vi "ClientForSingleDeviceDServer_03.vi"() -> ()   [LabVIEW 2014, in "examples.lvlib"]
uses:
  examples.lvlib
  Common/UtilsRandomInstances/_UtilsRandomI16Array.vi
  vis/tango_vi.llb/WriteShortSpectrumAttribute.vi
  vis/tango_vi.llb/ReadShortSpectrumAttribute.vi
  Common/UtilsRandomInstances/_UtilsRandomU16Array.vi
  vis/tango_vi.llb/WriteUShortSpectrumAttribute.vi
  vis/tango_vi.llb/ReadUShortSpectrumAttribute.vi
  Common/UtilsRandomInstances/_UtilsRandomBoolArray.vi
  vis/tango_vi.llb/WriteBooleanSpectrumAttribute.vi
  vis/tango_vi.llb/ReadBooleanSpectrumAttribute.vi
  Common/UtilsRandomInstances/_UtilsRandomU8Array.vi
  vis/tango_vi.llb/WriteUCharSpectrumAttribute.vi
  vis/tango_vi.llb/ReadUCharSpectrumAttribute.vi
  Common/UtilsRandomInstances/_UtilsRandom2DI16Array.vi
  vis/tango_vi.llb/WriteShortImageAttribute.vi
  vis/tango_vi.llb/ReadShortImageAttribute.vi
  Common/UtilsRandomInstances/_UtilsRandomSGLArray.vi
  vis/tango_vi.llb/WriteFloatSpectrumAttribute.vi
  vis/tango_vi.llb/ReadFloatSpectrumAttribute.vi
  Common/UtilsRandomInstances/_UtilsRandomDBLArray.vi
  vis/tango_vi.llb/WriteDoubleSpectrumAttribute.vi
  vis/tango_vi.llb/ReadDoubleSpectrumAttribute.vi
  Common/UtilsRandomInstances/_UtilsRandom2DI32Array.vi
  vis/tango_vi.llb/WriteLongImageAttribute.vi
  vis/tango_vi.llb/ReadLongImageAttribute.vi
  Common/UtilsRandomInstances/_UtilsRandomU32Array.vi
  vis/tango_vi.llb/WriteLongSpectrumAttribute.vi
  vis/tango_vi.llb/ReadLongSpectrumAttribute.vi
  Common/UtilsRandomInstances/_UtilsRandom2DU16Array.vi
  vis/tango_vi.llb/WriteUShortImageAttribute.vi
  vis/tango_vi.llb/ReadUShortImageAttribute.vi
  Common/UtilsRandomInstances/_UtilsRandom2DU8Array.vi
  vis/tango_vi.llb/WriteUCharImageAttribute.vi
  vis/tango_vi.llb/ReadUCharImageAttribute.vi
  Common/UtilsRandomInstances/_UtilsRandom2DBoolArray.vi
  vis/tango_vi.llb/WriteBooleanImageAttribute.vi
  vis/tango_vi.llb/ReadBooleanImageAttribute.vi
  Common/UtilsRandomInstances/_UtilsRandom2DSGLArray.vi
  vis/tango_vi.llb/WriteFloatImageAttribute.vi
  vis/tango_vi.llb/ReadFloatImageAttribute.vi
  Common/UtilsRandomInstances/_UtilsRandom2DDBLArray.vi
  vis/tango_vi.llb/WriteDoubleImageAttribute.vi
  vis/tango_vi.llb/ReadDoubleImageAttribute.vi
  Common/UtilsRandomInstances/_UtilsRandom2DU32Array.vi
  vis/tango_vi.llb/WriteULongImageAttribute.vi
  vis/tango_vi.llb/ReadULongImageAttribute.vi
  vis/tango_vi.llb/tango.lvlib
panel:
  out "Success-R":bool
  out "Success-Comp":bool
  out "devULongImage R":u32[][](graph)
  out "Success-W":bool
  out "devULongImage W":u32[][](graph)
  out "Success-R":bool
  out "Success-Comp":bool
  out "devDoubleImage R":dbl[][](graph)
  out "Success-W":bool
  out "devDoubleImage W":dbl[][](graph)
  out "Success-R":bool
  out "Success-Comp":bool
  out "devFloatImage R":sgl[][](graph)
  out "Success-W":bool
  out "devFloatImage W":sgl[][](graph)
  out "Success-R":bool
  out "Success-Comp":bool
  out "devBooleanImage R":i16[][](graph)
  out "Success-W":bool
  out "devBooleanImage W":i16[][](graph)
  out "Success-R":bool
  out "Success-Comp":bool
  out "devUCharImage R":u8[][](graph)
  out "Success-W":bool
  out "devUCharImage W":u8[][](graph)
  out "Success-R":bool
  out "Success-Comp":bool
  out "devUShortImage R":u16[][](graph)
  out "Success-W":bool
  out "devUShortImage W":u16[][](graph)
  out "devLongSpectrum R":i32[](graph)
  out "Success-R":bool
  out "Success-Comp":bool
  out "Success-W":bool
  out "devLongSpectrum W":i32[](graph)
  out "Success-R":bool
  out "Success-Comp":bool
  out "devLongImage R":i32[][](graph)
  out "Success-W":bool
  out "devLongImage W":i32[][](graph)
  out "devDoubleSpectrum R":dbl[](graph)
  out "Success-R":bool
  out "Success-Comp":bool
  out "Success-W":bool
  out "devDoubleSpectrum  W":dbl[](graph)
  out "devFloatSpectrum R":sgl[](graph)
  out "Success-R":bool
  out "Success-Comp":bool
  out "Success-W":bool
  out "devFloatSpectrum W":sgl[](graph)
  out "devShortImage R":i16[][](graph)
  out "devShortImage W":i16[][](graph)
  out "Success-R":bool
  out "Success-Comp":bool
  out "Success-W":bool
  in  "TangoTest Device Name 5":string="tango/tangotest/1"
  in  "TangoTest Device Name 4":string="tango/tangotest/1"
  in  "TangoTest Device Name 3":string="tango/tangotest/1"
  in  "TangoTest Device Name 2":string="tango/tangotest/1"
  in  "TangoTest dev. name":string="labview/device/1"
  out "devUCharSpectrum R":u8[](graph)
  out "Success-R":bool
  out "Success-Comp":bool
  out "Success-W":bool
  out "devUCharSpectrum W":u8[](graph)
  out "devBooleanSpectrum R":i16[](graph)
  out "Success-R":bool
  out "Success-Comp":bool
  out "Success-W":bool
  out "devBooleanSpectrum W":i16[](graph)
  out "devUShortSpectrum R":u16[](graph)
  out "Success-R":bool
  out "Success-Comp":bool
  out "Success-W":bool
  out "devUShortSpectrum W":u16[](graph)
  out "Success-Comp":bool
  out "Success-W":bool
  out "devShortSpectrum R":i16[](graph)
  out "Success-R":bool
  out "devShortSpectrum W":i16[](graph)
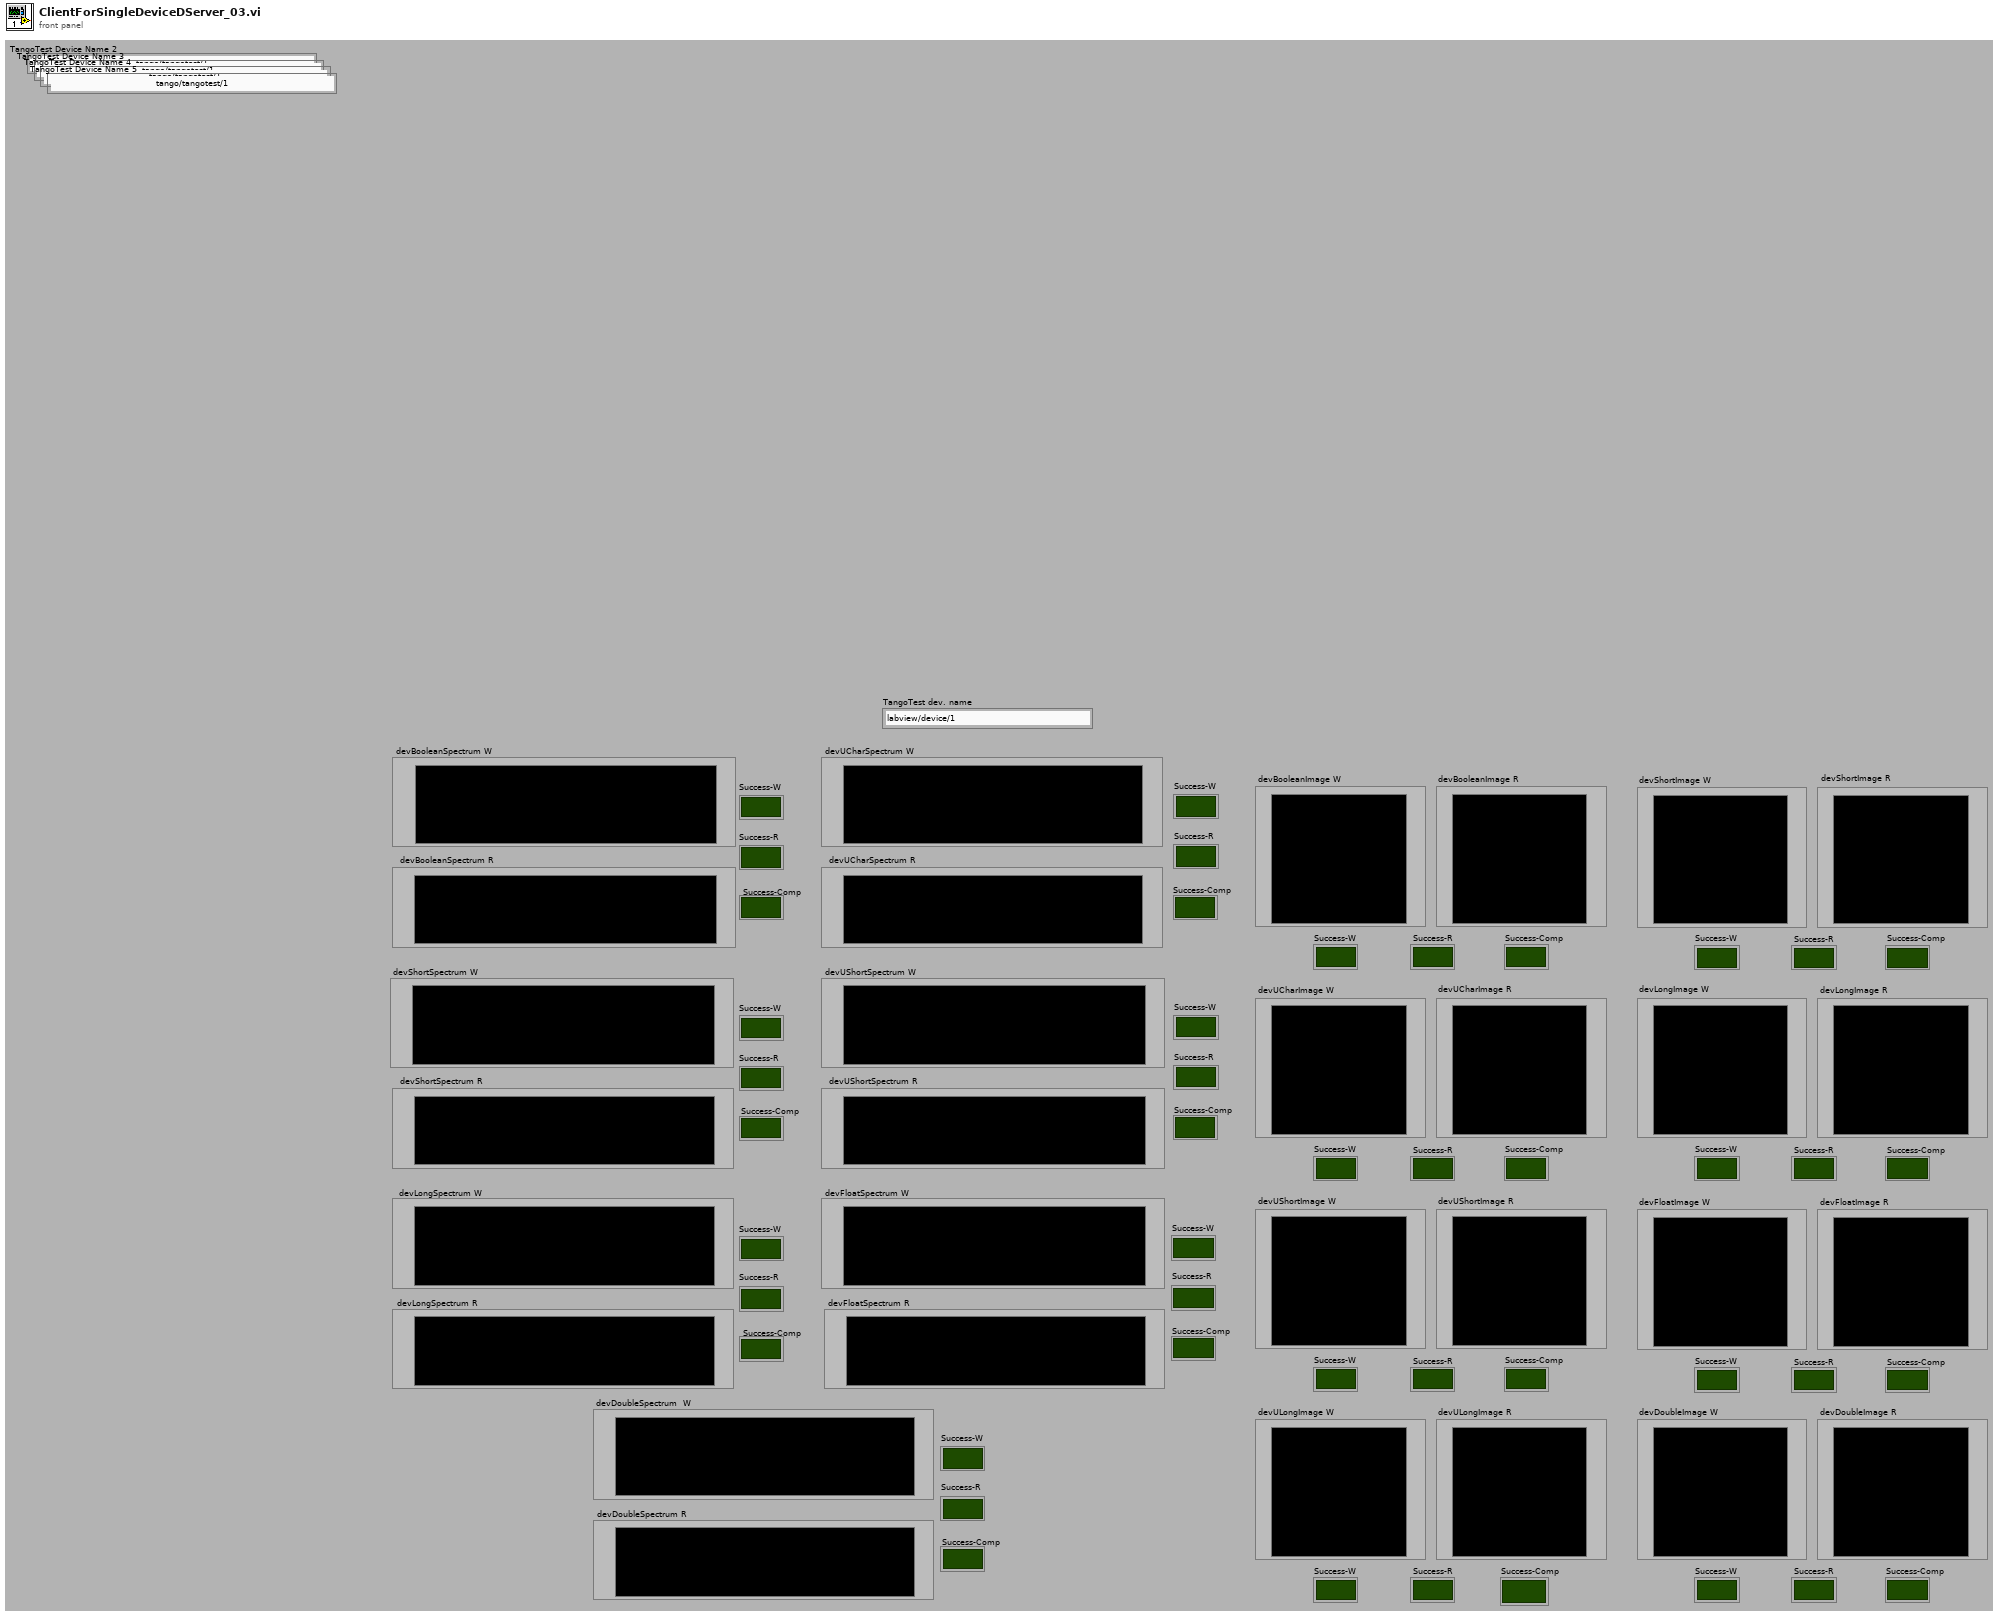
[diagram p1: front panel]
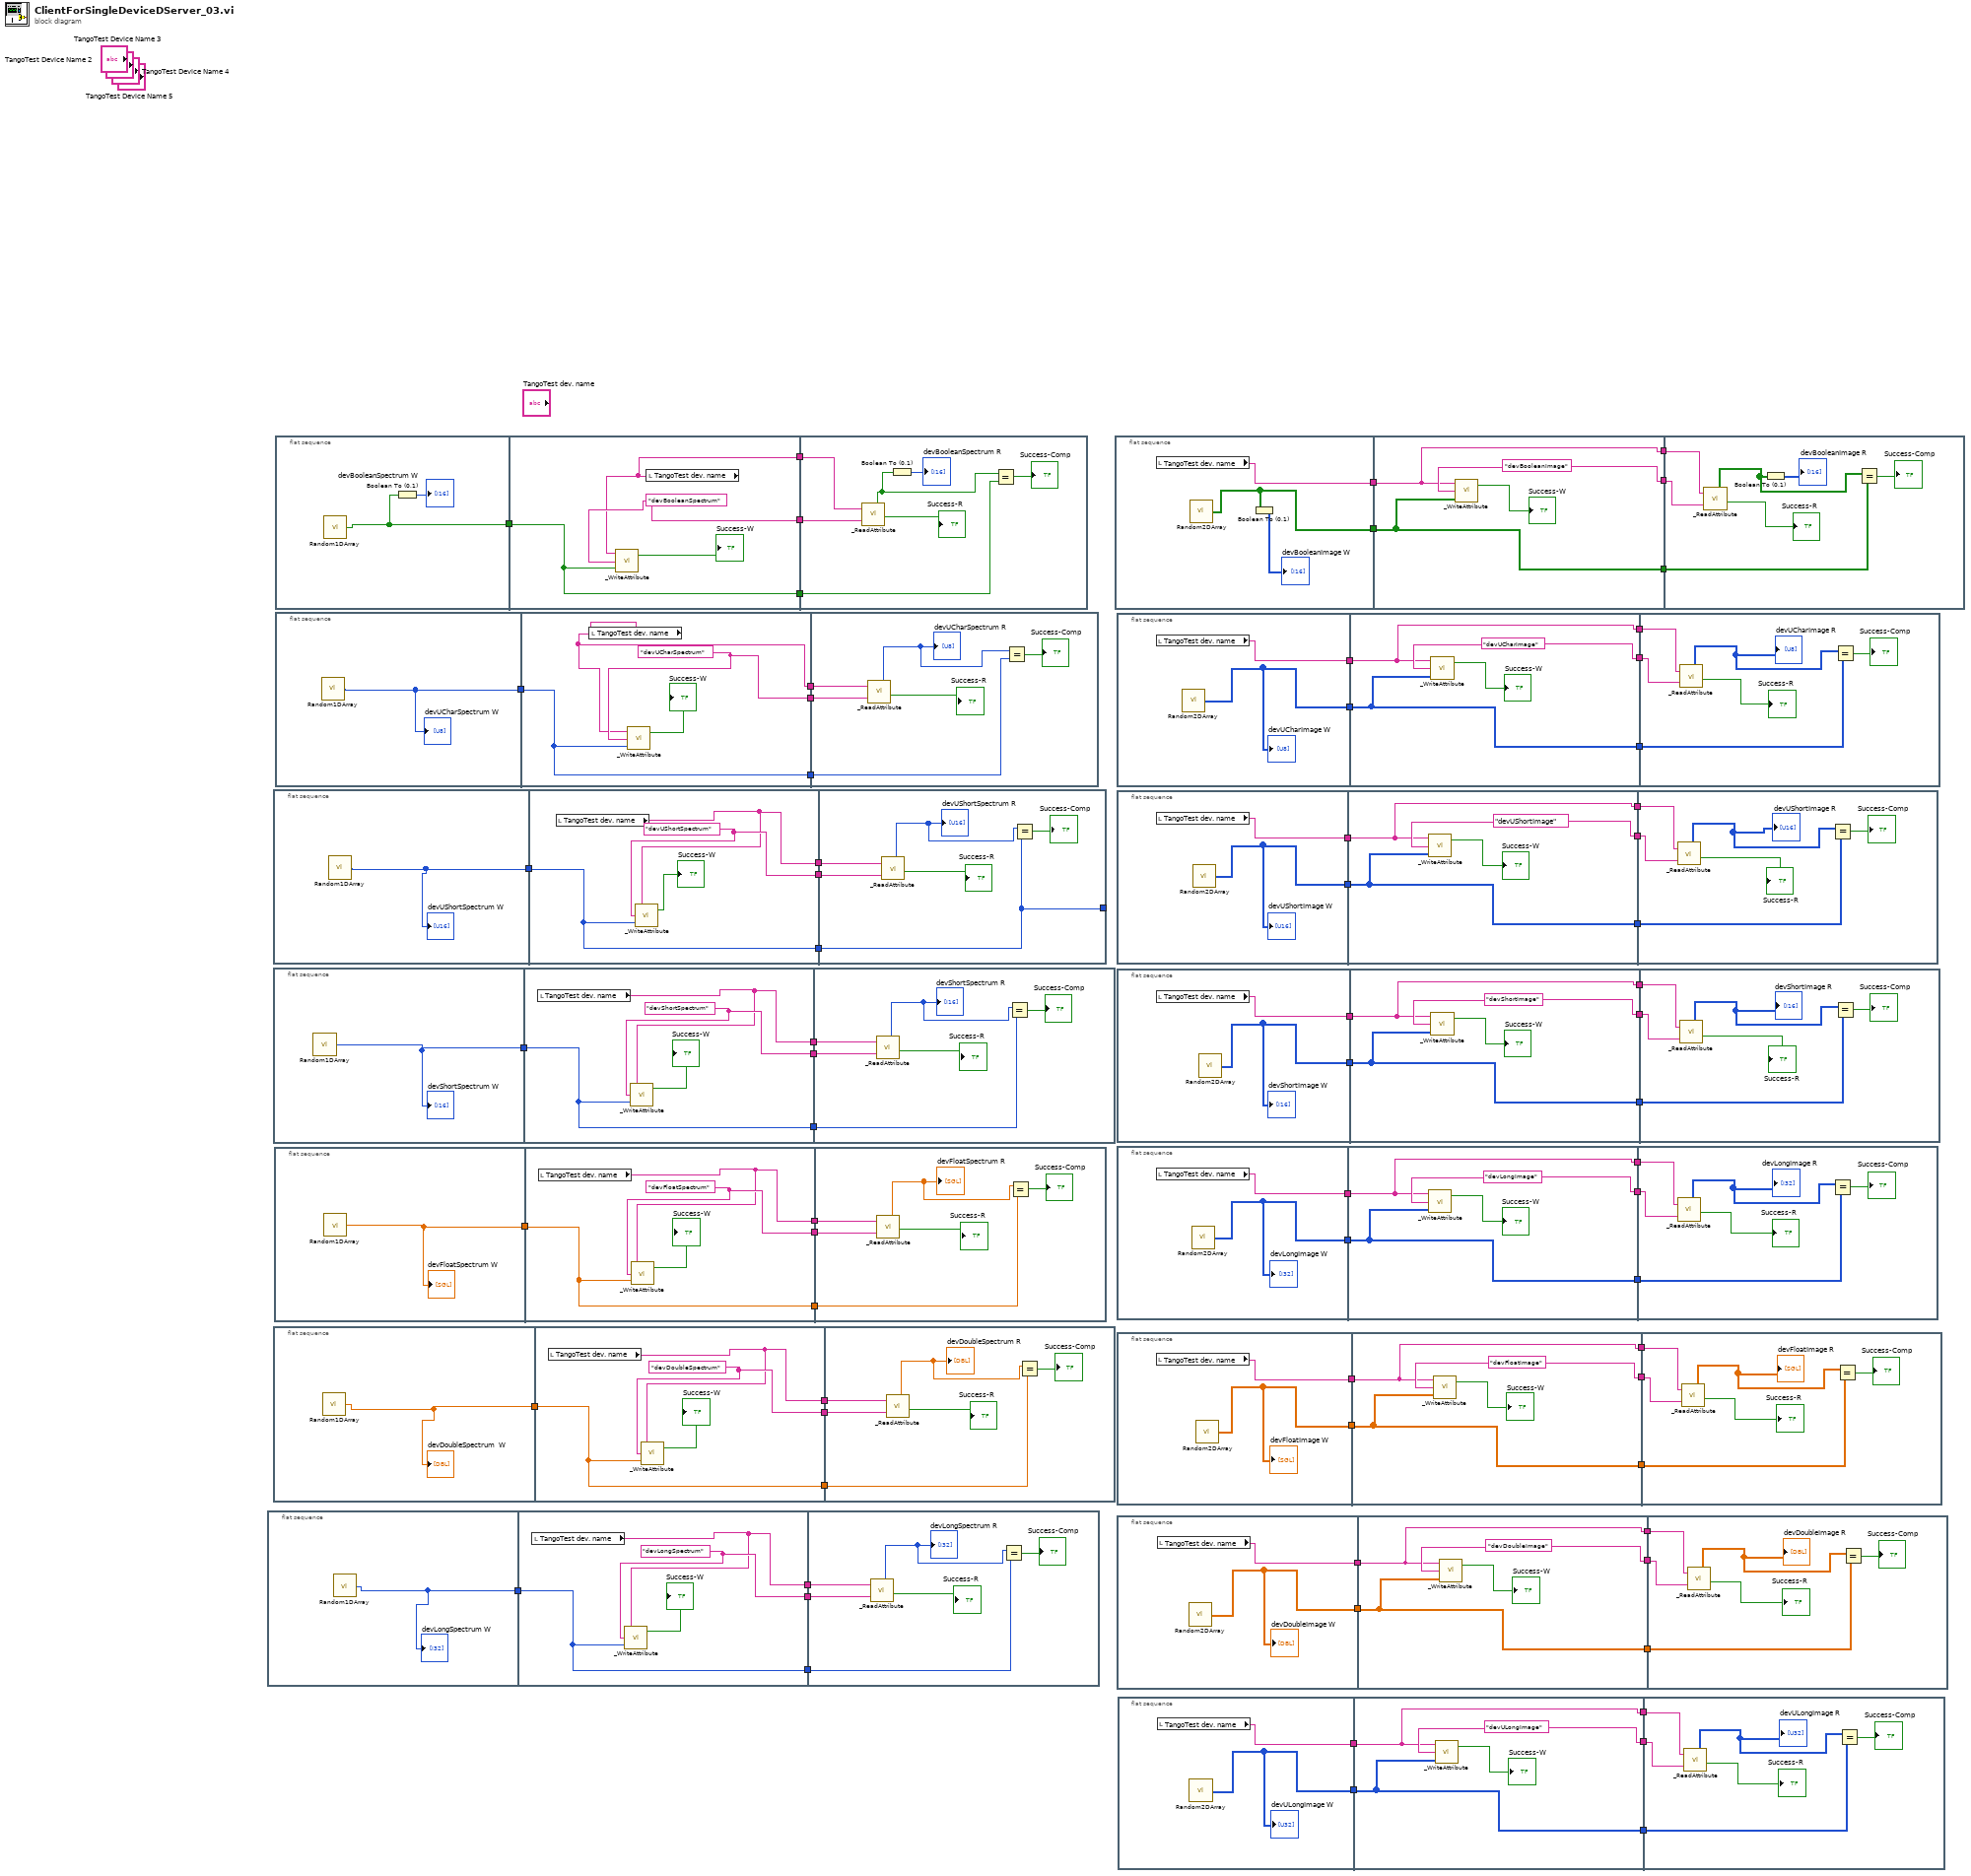
[diagram p0: block diagram]
diagram:
  n1 = flat-sequence {
    tunnel: [w69] -> w34
    tunnel: [w70] -> w33
    tunnel: [w72] -> w32
    tunnel: [w71] -> w31
    tunnel: w34 -> [w71]
    tunnel: w33 -> [w78]
    tunnel: w32 -> [w77]
    tunnel: w31 -> [w75]
    frame #0 {
      n2 = call-poly "Random1DArray.vi"() -> ("array"=w69:i32[])  [unwired: 2 in]
      "devLongSpectrum W" <- w69
    }
    frame #1 {
      w72 = "devLongSpectrum" ("attribute name")
      n3 = local read "TangoTest dev. name"() -> (w70:string)
      n4 = call-poly "_WriteAttribute.vi"("value"=w71, "attribute name"=w72, "device name"=w70) -> ("success"=→"Success-W":bool)  [unwired: 1 out]
    }
    frame #2 {
      n5 = call-poly "_ReadAttribute.vi"("device name"=w78, "attribute name"=w77) -> ("value"=w76:i32[], "success"=→"Success-R":bool)  [unwired: 4 out]
      "devLongSpectrum R" <- w76
      n6 = Equal?(x=w76, y=w75) -> (x = y?=→"Success-Comp":bool)
    }
  }
  n7 = flat-sequence {
    tunnel: [w80] -> w64
    tunnel: [w82] -> w63
    tunnel: [w84] -> w62
    tunnel: [w83] -> w61
    tunnel: w64 -> [w83]
    tunnel: w63 -> [w89]
    tunnel: w62 -> [w88]
    tunnel: w61 -> [w85]
    tunnel: [w85] -> _
    frame #0 {
      n8 = call-poly "Random1DArray.vi"() -> ("array"=w80:u16[])  [unwired: 2 in]
      "devUShortSpectrum W" <- w80
    }
    frame #1 {
      w84 = "devUShortSpectrum" ("attribute name")
      n9 = local read "TangoTest dev. name"() -> (w82:string)
      n10 = call-poly "_WriteAttribute.vi"("value"=w83, "attribute name"=w84, "device name"=w82) -> ("success"=→"Success-W":bool)  [unwired: 1 out]
    }
    frame #2 {
      n11 = call-poly "_ReadAttribute.vi"("device name"=w89, "attribute name"=w88) -> ("value"=w87:u16[], "success"=→"Success-R":bool)  [unwired: 4 out]
      "devUShortSpectrum R" <- w87
      n12 = Equal?(x=w87, y=w85) -> (x = y?=→"Success-Comp":bool)
    }
  }
  n13 = flat-sequence {
    tunnel: [w91] -> w65
    tunnel: [w92] -> w68
    tunnel: [w94] -> w67
    tunnel: [w93] -> w66
    tunnel: w65 -> [w93]
    tunnel: w68 -> [w100]
    tunnel: w67 -> [w99]
    tunnel: w66 -> [w97]
    frame #0 {
      n14 = call-poly "Random1DArray.vi"() -> ("array"=w91:i16[])  [unwired: 2 in]
      "devShortSpectrum W" <- w91
    }
    frame #1 {
      w94 = "devShortSpectrum" ("attribute name")
      n15 = local read "TangoTest dev. name"() -> (w92:string)
      n16 = call-poly "_WriteAttribute.vi"("value"=w93, "attribute name"=w94, "device name"=w92) -> ("success"=→"Success-W":bool)  [unwired: 1 out]
    }
    frame #2 {
      n17 = call-poly "_ReadAttribute.vi"("device name"=w100, "attribute name"=w99) -> ("value"=w98:i16[], "success"=→"Success-R":bool)  [unwired: 4 out]
      "devShortSpectrum R" <- w98
      n18 = Equal?(x=w98, y=w97) -> (x = y?=→"Success-Comp":bool)
    }
  }
  n19 = flat-sequence {
    tunnel: [w102] -> w43
    tunnel: [w103] -> w42
    tunnel: [w105] -> w41
    tunnel: [w104] -> w40
    tunnel: w43 -> [w104]
    tunnel: w42 -> [w111]
    tunnel: w41 -> [w110]
    tunnel: w40 -> [w108]
    frame #0 {
      n20 = call-poly "Random1DArray.vi"() -> ("array"=w102:dbl[])  [unwired: 2 in]
      "devDoubleSpectrum  W" <- w102
    }
    frame #1 {
      w105 = "devDoubleSpectrum" ("attribute name")
      n21 = local read "TangoTest dev. name"() -> (w103:string)
      n22 = call-poly "_WriteAttribute.vi"("value"=w104, "attribute name"=w105, "device name"=w103) -> ("success"=→"Success-W":bool)  [unwired: 1 out]
    }
    frame #2 {
      n23 = call-poly "_ReadAttribute.vi"("device name"=w111, "attribute name"=w110) -> ("value"=w109:dbl[], "success"=→"Success-R":bool)  [unwired: 4 out]
      "devDoubleSpectrum R" <- w109
      n24 = Equal?(x=w109, y=w108) -> (x = y?=→"Success-Comp":bool)
    }
  }
  n25 = flat-sequence {
    tunnel: [w113] -> w47
    tunnel: [w114] -> w46
    tunnel: [w116] -> w45
    tunnel: [w115] -> w44
    tunnel: w47 -> [w115]
    tunnel: w46 -> [w122]
    tunnel: w45 -> [w121]
    tunnel: w44 -> [w119]
    frame #0 {
      n26 = call-poly "Random1DArray.vi"() -> ("array"=w113:sgl[])  [unwired: 2 in]
      "devFloatSpectrum W" <- w113
    }
    frame #1 {
      w116 = "devFloatSpectrum" ("attribute name")
      n27 = local read "TangoTest dev. name"() -> (w114:string)
      n28 = call-poly "_WriteAttribute.vi"("value"=w115, "attribute name"=w116, "device name"=w114) -> ("success"=→"Success-W":bool)  [unwired: 1 out]
    }
    frame #2 {
      n29 = call-poly "_ReadAttribute.vi"("device name"=w122, "attribute name"=w121) -> ("value"=w120:sgl[], "success"=→"Success-R":bool)  [unwired: 4 out]
      "devFloatSpectrum R" <- w120
      n30 = Equal?(x=w120, y=w119) -> (x = y?=→"Success-Comp":bool)
    }
  }
  n31 = flat-sequence {
    tunnel: [w124] -> w54
    tunnel: [w125] -> w58
    tunnel: [w127] -> w57
    tunnel: w54 -> [w126]
    tunnel: [w126] -> w53
    tunnel: w58 -> [w133]
    tunnel: w57 -> [w132]
    tunnel: w53 -> [w129]
    frame #0 {
      n32 = call-poly "Random1DArray.vi"() -> ("array"=w124:u8[])  [unwired: 2 in]
      "devUCharSpectrum W" <- w124
    }
    frame #1 {
      w127 = "devUCharSpectrum" ("attribute name")
      n33 = local read "TangoTest dev. name"() -> (w125:string)
      n34 = call-poly "_WriteAttribute.vi"("value"=w126, "attribute name"=w127, "device name"=w125) -> ("success"=→"Success-W":bool)  [unwired: 1 out]
    }
    frame #2 {
      n35 = call-poly "_ReadAttribute.vi"("device name"=w133, "attribute name"=w132) -> ("value"=w131:u8[], "success"=→"Success-R":bool)  [unwired: 4 out]
      "devUCharSpectrum R" <- w131
      n36 = Equal?(x=w131, y=w129) -> (x = y?=→"Success-Comp":bool)
    }
  }
  n37 = flat-sequence {
    tunnel: [w135] -> w60
    tunnel: [w139] -> w59
    tunnel: w60 -> [w139]
    tunnel: [w138] -> w56
    tunnel: [w137] -> w55
    tunnel: w59 -> [w143]
    tunnel: w56 -> [w142]
    tunnel: w55 -> [w141]
    frame #0 {
      n38 = call-poly "Random1DArray.vi"() -> ("array"=w135:bool[])  [unwired: 2 in]
      n39 = Boolean To (0,1)(Boolean=w135) -> (0, 1=→"devBooleanSpectrum W":i16[])
    }
    frame #1 {
      w138 = "devBooleanSpectrum" ("attribute name")
      n40 = local read "TangoTest dev. name"() -> (w137:string)
      n41 = call-poly "_WriteAttribute.vi"("value"=w139, "attribute name"=w138, "device name"=w137) -> ("success"=→"Success-W":bool)  [unwired: 1 out]
    }
    frame #2 {
      n42 = call-poly "_ReadAttribute.vi"("device name"=w141, "attribute name"=w142) -> ("value"=w145:bool[], "success"=→"Success-R":bool)  [unwired: 4 out]
      n43 = Boolean To (0,1)(Boolean=w145) -> (0, 1=→"devBooleanSpectrum R":i16[])
      n44 = Equal?(x=w145, y=w143) -> (x = y?=→"Success-Comp":bool)
    }
  }
  n45 = flat-sequence {
    tunnel: [w148] -> w20
    tunnel: [w150] -> w19
    tunnel: [w154] -> w18
    tunnel: [w152] -> w17
    tunnel: w20 -> [w152]
    tunnel: w19 -> [w151]
    tunnel: [w151] -> w16
    tunnel: w18 -> [w160]
    tunnel: w17 -> [w157]
    tunnel: w16 -> [w156]
    frame #0 {
      n46 = local read "TangoTest dev. name"() -> (w150:string)
      n47 = call-poly "Random2DArray.vi"() -> ("random array"=w148:bool[][])  [unwired: 2 in]
      n48 = Boolean To (0,1)(Boolean=w148) -> (0, 1=→"devBooleanImage W":i16[][])
    }
    frame #1 {
      w154 = "devBooleanImage" ("attribute name")
      n49 = call-poly "_WriteAttribute.vi"("value"=w152, "attribute name"=w154, "device name"=w151) -> ("success"=→"Success-W":bool)  [unwired: 1 out]
    }
    frame #2 {
      n50 = call-poly "_ReadAttribute.vi"("device name"=w156, "attribute name"=w160) -> ("value"=w158:bool[][], "success"=→"Success-R":bool)  [unwired: 4 out]
      n51 = Boolean To (0,1)(Boolean=w158) -> (0, 1=→"devBooleanImage R":i16[][])
      n52 = Equal?(x=w158, y=w157) -> (x = y?=→"Success-Comp":bool)
    }
  }
  n53 = flat-sequence {
    tunnel: [w162] -> w25
    tunnel: [w163] -> w24
    tunnel: [w167] -> w23
    tunnel: [w165] -> w22
    tunnel: w25 -> [w165]
    tunnel: w24 -> [w164]
    tunnel: [w164] -> w21
    tunnel: w23 -> [w172]
    tunnel: w22 -> [w169]
    tunnel: w21 -> [w168]
    frame #0 {
      n54 = local read "TangoTest dev. name"() -> (w163:string)
      n55 = call-poly "Random2DArray.vi"() -> ("random array"=w162:u8[][])  [unwired: 2 in]
      "devUCharImage W" <- w162
    }
    frame #1 {
      w167 = "devUCharImage" ("attribute name")
      n56 = call-poly "_WriteAttribute.vi"("value"=w165, "attribute name"=w167, "device name"=w164) -> ("success"=→"Success-W":bool)  [unwired: 1 out]
    }
    frame #2 {
      n57 = call-poly "_ReadAttribute.vi"("device name"=w168, "attribute name"=w172) -> ("value"=w170:u8[][], "success"=→"Success-R":bool)  [unwired: 4 out]
      "devUCharImage R" <- w170
      n58 = Equal?(x=w170, y=w169) -> (x = y?=→"Success-Comp":bool)
    }
  }
  n59 = flat-sequence {
    tunnel: [w174] -> w30
    tunnel: [w175] -> w29
    tunnel: [w179] -> w28
    tunnel: [w177] -> w27
    tunnel: w30 -> [w177]
    tunnel: w29 -> [w176]
    tunnel: [w176] -> w26
    tunnel: w28 -> [w184]
    tunnel: w27 -> [w182]
    tunnel: w26 -> [w181]
    frame #0 {
      n60 = local read "TangoTest dev. name"() -> (w175:string)
      n61 = call-poly "Random2DArray.vi"() -> ("random array"=w174:u16[][])  [unwired: 2 in]
      "devUShortImage W" <- w174
    }
    frame #1 {
      w179 = "devUShortImage" ("attribute name")
      n62 = call-poly "_WriteAttribute.vi"("value"=w177, "attribute name"=w179, "device name"=w176) -> ("success"=→"Success-W":bool)  [unwired: 1 out]
    }
    frame #2 {
      n63 = call-poly "_ReadAttribute.vi"("device name"=w181, "attribute name"=w184) -> ("value"=w180:u16[][], "success"=→"Success-R":bool)  [unwired: 4 out]
      "devUShortImage R" <- w180
      n64 = Equal?(x=w180, y=w182) -> (x = y?=→"Success-Comp":bool)
    }
  }
  n65 = flat-sequence {
    tunnel: [w187] -> w50
    tunnel: [w186] -> w49
    tunnel: [w191] -> w52
    tunnel: [w189] -> w51
    tunnel: w50 -> [w189]
    tunnel: w49 -> [w188]
    tunnel: [w188] -> w48
    tunnel: w52 -> [w196]
    tunnel: w51 -> [w193]
    tunnel: w48 -> [w192]
    frame #0 {
      n66 = local read "TangoTest dev. name"() -> (w186:string)
      n67 = call-poly "Random2DArray.vi"() -> ("random array"=w187:i16[][])  [unwired: 2 in]
      "devShortImage W" <- w187
    }
    frame #1 {
      w191 = "devShortImage" ("attribute name")
      n68 = call-poly "_WriteAttribute.vi"("value"=w189, "attribute name"=w191, "device name"=w188) -> ("success"=→"Success-W":bool)  [unwired: 1 out]
    }
    frame #2 {
      n69 = call-poly "_ReadAttribute.vi"("device name"=w192, "attribute name"=w196) -> ("value"=w194:i16[][], "success"=→"Success-R":bool)  [unwired: 4 out]
      "devShortImage R" <- w194
      n70 = Equal?(x=w194, y=w193) -> (x = y?=→"Success-Comp":bool)
    }
  }
  n71 = flat-sequence {
    tunnel: [w198] -> w39
    tunnel: [w199] -> w38
    tunnel: [w203] -> w37
    tunnel: [w201] -> w36
    tunnel: w39 -> [w201]
    tunnel: w38 -> [w200]
    tunnel: [w200] -> w35
    tunnel: w37 -> [w208]
    tunnel: w36 -> [w205]
    tunnel: w35 -> [w204]
    frame #0 {
      n72 = local read "TangoTest dev. name"() -> (w199:string)
      n73 = call-poly "Random2DArray.vi"() -> ("random array"=w198:i32[][])  [unwired: 2 in]
      "devLongImage W" <- w198
    }
    frame #1 {
      w203 = "devLongImage" ("attribute name")
      n74 = call-poly "_WriteAttribute.vi"("value"=w201, "attribute name"=w203, "device name"=w200) -> ("success"=→"Success-W":bool)  [unwired: 1 out]
    }
    frame #2 {
      n75 = call-poly "_ReadAttribute.vi"("device name"=w204, "attribute name"=w208) -> ("value"=w206:i32[][], "success"=→"Success-R":bool)  [unwired: 4 out]
      "devLongImage R" <- w206
      n76 = Equal?(x=w206, y=w205) -> (x = y?=→"Success-Comp":bool)
    }
  }
  n77 = flat-sequence {
    tunnel: [w210] -> w15
    tunnel: [w211] -> w14
    tunnel: [w215] -> w13
    tunnel: [w213] -> w12
    tunnel: w15 -> [w213]
    tunnel: w14 -> [w212]
    tunnel: [w212] -> w11
    tunnel: w13 -> [w220]
    tunnel: w12 -> [w217]
    tunnel: w11 -> [w216]
    frame #0 {
      n78 = local read "TangoTest dev. name"() -> (w211:string)
      n79 = call-poly "Random2DArray.vi"() -> ("random array"=w210:sgl[][])  [unwired: 2 in]
      "devFloatImage W" <- w210
    }
    frame #1 {
      w215 = "devFloatImage" ("attribute name")
      n80 = call-poly "_WriteAttribute.vi"("value"=w213, "attribute name"=w215, "device name"=w212) -> ("success"=→"Success-W":bool)  [unwired: 1 out]
    }
    frame #2 {
      n81 = call-poly "_ReadAttribute.vi"("device name"=w216, "attribute name"=w220) -> ("value"=w218:sgl[][], "success"=→"Success-R":bool)  [unwired: 4 out]
      "devFloatImage R" <- w218
      n82 = Equal?(x=w218, y=w217) -> (x = y?=→"Success-Comp":bool)
    }
  }
  n83 = flat-sequence {
    tunnel: [w222] -> w10
    tunnel: [w223] -> w9
    tunnel: [w227] -> w8
    tunnel: [w225] -> w7
    tunnel: w10 -> [w225]
    tunnel: w9 -> [w224]
    tunnel: [w224] -> w6
    tunnel: w8 -> [w232]
    tunnel: w7 -> [w229]
    tunnel: w6 -> [w228]
    frame #0 {
      n84 = local read "TangoTest dev. name"() -> (w223:string)
      n85 = call-poly "Random2DArray.vi"() -> ("random array"=w222:dbl[][])  [unwired: 2 in]
      "devDoubleImage W" <- w222
    }
    frame #1 {
      w227 = "devDoubleImage" ("attribute name")
      n86 = call-poly "_WriteAttribute.vi"("value"=w225, "attribute name"=w227, "device name"=w224) -> ("success"=→"Success-W":bool)  [unwired: 1 out]
    }
    frame #2 {
      n87 = call-poly "_ReadAttribute.vi"("device name"=w228, "attribute name"=w232) -> ("value"=w230:dbl[][], "success"=→"Success-R":bool)  [unwired: 4 out]
      "devDoubleImage R" <- w230
      n88 = Equal?(x=w230, y=w229) -> (x = y?=→"Success-Comp":bool)
    }
  }
  n89 = flat-sequence {
    tunnel: [w234] -> w5
    tunnel: [w235] -> w4
    tunnel: [w239] -> w3
    tunnel: [w237] -> w2
    tunnel: w5 -> [w237]
    tunnel: w4 -> [w236]
    tunnel: [w236] -> w1
    tunnel: w3 -> [w244]
    tunnel: w2 -> [w241]
    tunnel: w1 -> [w240]
    frame #0 {
      n90 = local read "TangoTest dev. name"() -> (w235:string)
      n91 = call-poly "Random2DArray.vi"() -> ("random array"=w234:u32[][])  [unwired: 2 in]
      "devULongImage W" <- w234
    }
    frame #1 {
      w239 = "devULongImage" ("attribute name")
      n92 = call-poly "_WriteAttribute.vi"("value"=w237, "attribute name"=w239, "device name"=w236) -> ("success"=→"Success-W":bool)  [unwired: 1 out]
    }
    frame #2 {
      n93 = call-poly "_ReadAttribute.vi"("device name"=w240, "attribute name"=w244) -> ("value"=w242:u32[][], "success"=→"Success-R":bool)  [unwired: 4 out]
      "devULongImage R" <- w242
      n94 = Equal?(x=w242, y=w241) -> (x = y?=→"Success-Comp":bool)
    }
  }
